vi "102-3102-report5-gaydos.vi"() -> ()   [LabVIEW 2011]
uses:
  <vilib>/imath/engines/lvmath2/RunTimeEngine/ErrorHandling/NIMS_Finalize Error.vi
  <vilib>/imath/engines/lvmath2/RunTimeEngine/Managers/WorkSpace/UID Generator.vi
  <vilib>/imath/engines/lvmath2/RunTimeEngine/Managers/SymbolTable/Clear UID.vi
  <vilib>/imath/engines/lvmath2/RunTimeEngine/NodeEndStatement/NIMS_NodeEndStatement_Output.vi
  <instcachedir>/0/NIMS_NodeEndStatement_Output_53EC0D466D134D7ABD903AC30B43404B.lvgen/NIMS_NodeEndStatement_Output_53EC0D466D134D7ABD903AC30B43404B_005.vi
  <instcachedir>/0/NIMS_NodeEndStatement_Output_53EC0D466D134D7ABD903AC30B43404B.lvgen/NIMS_NodeEndStatement_Output_53EC0D466D134D7ABD903AC30B43404B_000.vi
  <instcachedir>/0/NIMS_NodeEndStatement_Output_53EC0D466D134D7ABD903AC30B43404B.lvgen/NIMS_NodeEndStatement_Output_53EC0D466D134D7ABD903AC30B43404B_001.vi
  <instcachedir>/0/NIMS_NodeEndStatement_Output_53EC0D466D134D7ABD903AC30B43404B.lvgen/NIMS_NodeEndStatement_Output_53EC0D466D134D7ABD903AC30B43404B_004.vi
  <vilib>/imath/engines/lvmath2/RunTimeEngine/RangeToken/NIMS_Range.vi
  <instcachedir>/0/NIMS_Range_0B7635FB69F84E19AA68E7FF959DF37C.lvgen/NIMS_Range_0B7635FB69F84E19AA68E7FF959DF37C_001.vi
  <vilib>/imath/engines/lvmath2/RunTimeEngine/RunTimeType/NIMS_RunTimeType_From StrictType (excl LVString).vi
  <instcachedir>/0/NIMS_RunTimeType_From StrictType (excl LVString)_46AE8B54A11948F0BCCEB8091EE7AA4C.lvgen/NIMS_RunTimeType_From StrictType (excl LVString)_46AE8B54A11948F0BCCEB8091EE7AA4C_000.vi
  <vilib>/imathl/engines/lvmath/Functions/Error Handling/Create Error.vi
  <vilib>/imath/engines/lvmath2/RunTimeEngine/LocalVariableDefStatement/MC_LocalVariableDefStatement_Display.vi
  <vilib>/imath/engines/lvmath2/RunTimeEngine/BuiltInFunctions/zeros/NIMS_V=zeros(I32,I32).vi
  <vilib>/imath/engines/lvmath2/RunTimeEngine/BuiltInFunctions/ones/NIMS_V=ones(I32,I32).vi
  <vilib>/imath/engines/lvmath2/RunTimeEngine/ErrorHandling/NIMS_Create Error From Enums.vi
  <vilib>/imath/engines/lvmath2/RunTimeEngine/BuiltInFunctions/conv/NIMS_conv(V,V).vi
  <instcachedir>/0/NIMS_conv(V,V)_D3E194F2B5174935BB2368CEB7AAC5A9.lvgen/NIMS_conv(V,V)_D3E194F2B5174935BB2368CEB7AAC5A9_000.vi
  <vilib>/imath/engines/lvmath2/RunTimeEngine/ErrorHandling/NIMS_Error From Error Code.vi
  <vilib>/imath/engines/lvmath2/RunTimeEngine/BuiltInFunctions/fft/NIMS_fft(GV).vi
  <instcachedir>/0/NIMS_fft(GV)_4C6467FC22F84E4BA42517A07EF978B0.lvgen/NIMS_fft(GV)_4C6467FC22F84E4BA42517A07EF978B0_000.vi
  <vilib>/imath/engines/lvmath2/RunTimeEngine/BuiltInFunctions/fftshift/NIMS_fftshift(GV).vi
  <instcachedir>/0/NIMS_fftshift(GV)_BD7A7BA9CA6B470B9A9F73A6A3FEEB3E.lvgen/NIMS_fftshift(GV)_BD7A7BA9CA6B470B9A9F73A6A3FEEB3E_000.vi
  <vilib>/imath/engines/lvmath2/RunTimeEngine/ArithmeticOperatorToken/NIMS_ArithmeticOperator_times.vi
  <instcachedir>/0/NIMS_ArithmeticOperator_times_3FA9DDB491BD45F6905798C0465C9825.lvgen/NIMS_ArithmeticOperator_times_3FA9DDB491BD45F6905798C0465C9825_003.vi
  <instcachedir>/0/NIMS_fft(GV)_4C6467FC22F84E4BA42517A07EF978B0.lvgen/NIMS_fft(GV)_4C6467FC22F84E4BA42517A07EF978B0_001.vi
  <vilib>/imath/engines/lvmath2/RunTimeEngine/BuiltInFunctions/ifft_shift/NIMS_ifft_shift(GV).vi
  <instcachedir>/0/NIMS_ifft_shift(GV)_21661D804B78421B969BCA642CA10C0F.lvgen/NIMS_ifft_shift(GV)_21661D804B78421B969BCA642CA10C0F_000.vi
  <vilib>/imath/engines/lvmath2/RunTimeEngine/BuiltInFunctions/ifft/NIMS_ifft(CV).vi
  <vilib>/imath/engines/lvmath2/RunTimeEngine/BuiltInFunctions/length/NIMS_length(GV).vi
  <instcachedir>/0/NIMS_length(GV)_08A3D13377FD4E4B96F5795FBF3698FA.lvgen/NIMS_length(GV)_08A3D13377FD4E4B96F5795FBF3698FA_002.vi
  <vilib>/imath/engines/lvmath2/RunTimeEngine/BuiltInFunctions/abs/NIMS_abs(signed).vi
  <instcachedir>/0/NIMS_abs(signed)_C4FCB8E6058B49B797C7C8D53CA5F6EC.lvgen/NIMS_abs(signed)_C4FCB8E6058B49B797C7C8D53CA5F6EC_006.vi
  <vilib>/imath/engines/lvmath2/RunTimeEngine/BuiltInFunctions/angle/NIMS_angle.vi
  <instcachedir>/0/NIMS_angle_6DDAE2BD99E0421EB990B6436E94D88F.lvgen/NIMS_angle_6DDAE2BD99E0421EB990B6436E94D88F_002.vi
  <vilib>/imath/engines/lvmath2/RunTimeEngine/Managers/SymbolTable/NIMS_WorkSpace.lvlib
panel:
  out "Phase of H(jw)":cluster{"Y":dbl[], "Y":dbl[]}[](graph)
  out "Magnitude of H(jw)":cluster{"Y":dbl[], "Y":dbl[]}[](graph)
  out "Phase of X(jw)":cluster{"Y":dbl[], "Y":dbl[]}[](graph)
  out "Magnitude of X(jw)":cluster{"Y":dbl[], "Y":dbl[]}[](graph)
  out "Phase of Y(jw)":cluster{"Y":dbl[], "Y":dbl[]}[](graph)
  out "Magnitude of Y(jw)":cluster{"Y":dbl[], "Y":dbl[]}[](graph)
  out "y(t) and ift of y(t)":dynamicdata(graph)
  out "h(t)":waveform(dbl)(graph)
  out "x(t)":waveform(i32)(graph)
  in  "D":dbl
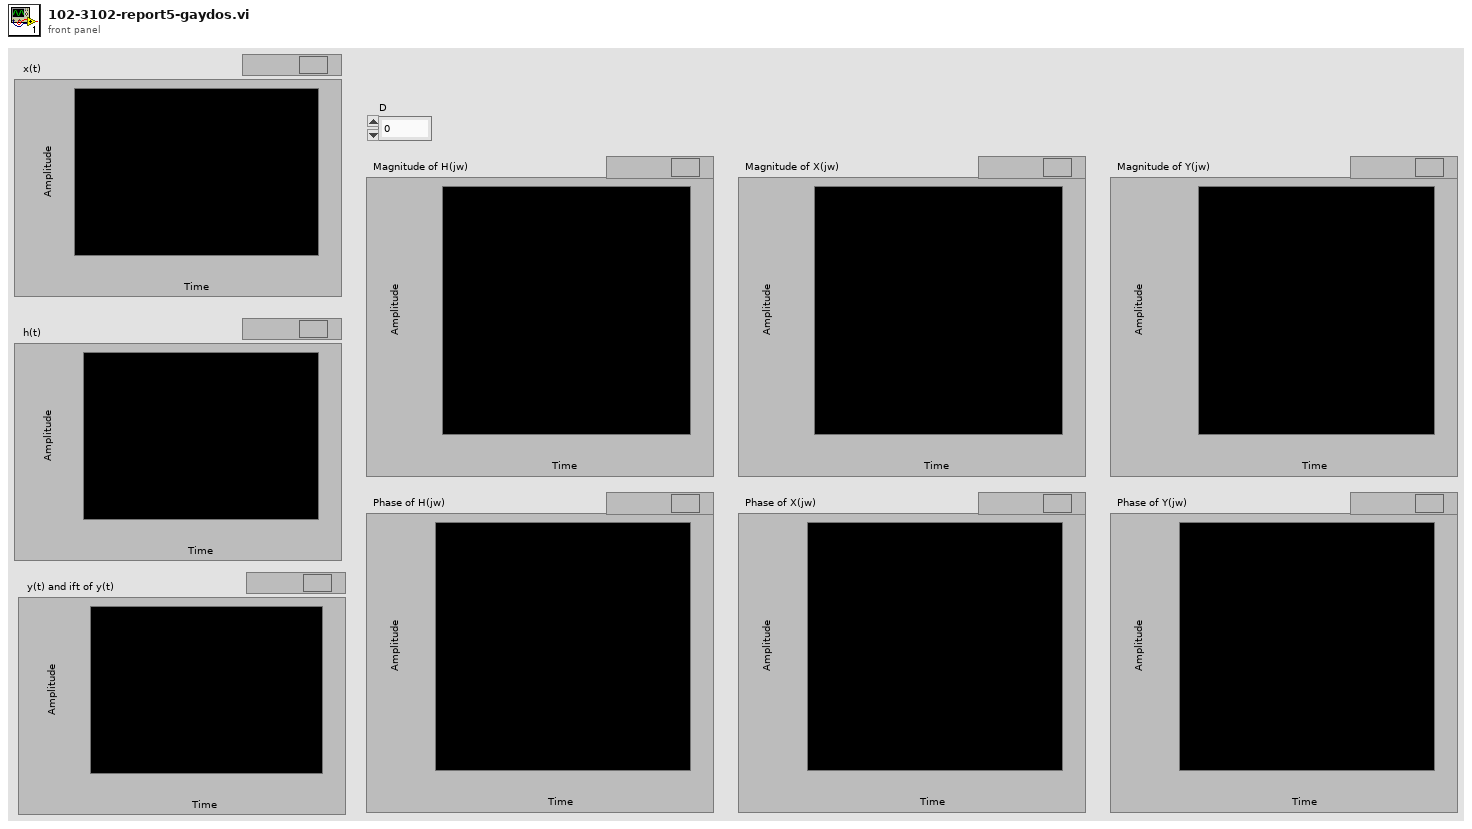
[diagram p1: front panel]
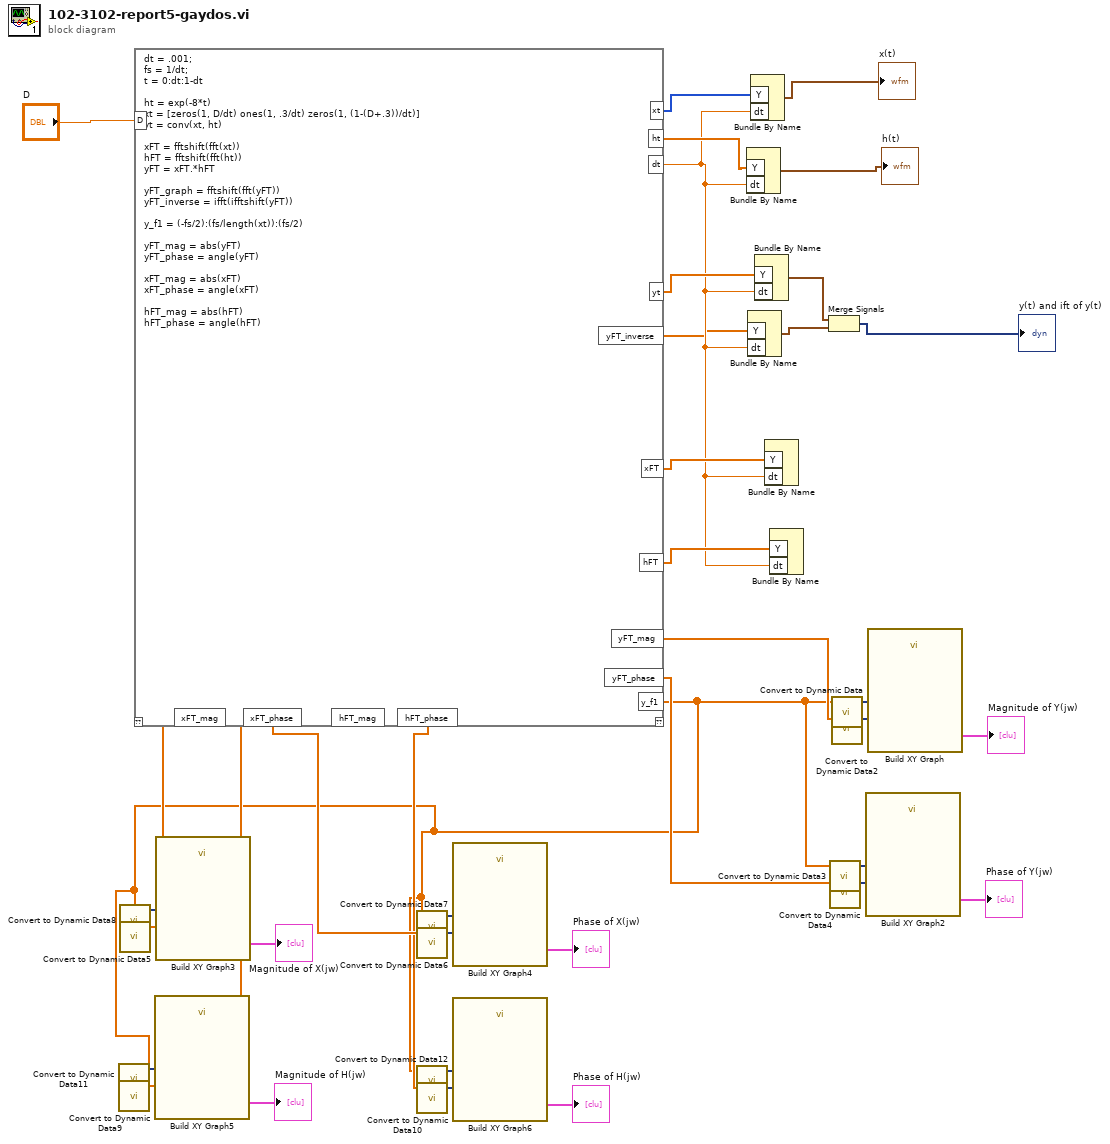
[diagram p0: block diagram]
diagram:
  n1 = mathscript code="dt = .001;\nfs = 1/dt;\nt = 0:dt:1-dt\n\nht = exp(-8*t)\nxt = [zeros(1, D/dt) ones(1, .3/dt) zeros(1, (1-(D+.3))/dt)]\nyt = conv(xt, ht)\n\nxFT = fftshift(fft(xt))\nhFT = fftshift(fft(ht))\nyFT = xFT.*hFT\n\nyFT_graph = fftshift(fft(yFT))\nyFT_inverse = ifft(ifftshift(yFT))\n\ny_f1 = (-fs/2):(fs/length(xt)):(fs/2)\n\nyFT_mag = abs(yFT)\nyFT_phase = angle(yFT)\n\nxFT_mag = abs(xFT)\nxFT_phase = angle(xFT)\n\nhFT_mag = abs(hFT)\nhFT_phase = angle(hFT)"("D"="D") -> ("xt"=w37:i32[], "ht"=w36:dbl[], "dt"=w28:dbl, "yt"=w33:dbl[], "hFT"=w29:cdb[], "xFT"=w30:cdb[], "yFT_mag"=w19:dbl[], "yFT_phase"=w18:dbl[], "yFT_inverse"=w26:dbl[], "y_f1"=w2:dbl[], "xFT_mag"=w15:dbl[], "xFT_phase"=w13:dbl[], "hFT_mag"=w7:dbl[], "hFT_phase"=w5:dbl[])  [unwired: 1 in, 1 out]
  n2 = call "Convert to Dynamic Data11"("Array"=w2) -> ("Dynamic Data Type"=w3:dynamicdata)  [unwired: 3 in]
  n3 = call "Convert to Dynamic Data9"("Array"=w7) -> ("Dynamic Data Type"=w6:dynamicdata)  [unwired: 3 in]
  n4 = call "Convert to Dynamic Data8"("Array"=w2) -> ("Dynamic Data Type"=w10:dynamicdata)  [unwired: 3 in]
  n5 = call "Convert to Dynamic Data5"("Array"=w15) -> ("Dynamic Data Type"=w14:dynamicdata)  [unwired: 3 in]
  n6 = call "Build XY Graph5"("Y Input"=w6, "X Input"=w3) -> ("XY Graph"=→"Magnitude of H(jw)":cluster{"Y":dbl[], "Y":dbl[]}[])  [unwired: 3 in, 6 out]
  n7 = call "Build XY Graph3"("Y Input"=w14, "X Input"=w10) -> ("XY Graph"=→"Magnitude of X(jw)":cluster{"Y":dbl[], "Y":dbl[]}[])  [unwired: 3 in, 6 out]
  n8 = call "Convert to Dynamic Data7"("Array"=w2) -> ("Dynamic Data Type"=w11:dynamicdata)  [unwired: 3 in]
  n9 = call "Convert to Dynamic Data6"("Array"=w13) -> ("Dynamic Data Type"=w12:dynamicdata)  [unwired: 3 in]
  n10 = call "Convert to Dynamic Data12"("Array"=w2) -> ("Dynamic Data Type"=w1:dynamicdata)  [unwired: 3 in]
  n11 = call "Convert to Dynamic Data10"("Array"=w5) -> ("Dynamic Data Type"=w4:dynamicdata)  [unwired: 3 in]
  n12 = call "Build XY Graph4"("Y Input"=w12, "X Input"=w11) -> ("XY Graph"=→"Phase of X(jw)":cluster{"Y":dbl[], "Y":dbl[]}[])  [unwired: 3 in, 6 out]
  n13 = call "Build XY Graph6"("Y Input"=w4, "X Input"=w1) -> ("XY Graph"=→"Phase of H(jw)":cluster{"Y":dbl[], "Y":dbl[]}[])  [unwired: 3 in, 6 out]
  n14 = Bundle By Name("Y"=w36, "dt"=w28) -> (→"h(t)":waveform(dbl))  [unwired: 1 in]
  n15 = Bundle By Name("Y"=w26, "dt"=w28) -> (w25:waveform(dbl))  [unwired: 1 in]
  n16 = Bundle By Name("Y"=w37, "dt"=w28) -> (→"x(t)":waveform(i32))  [unwired: 1 in]
  n17 = Bundle By Name("Y"=w33, "dt"=w28) -> (w32:waveform(dbl))  [unwired: 1 in]
  n18 = Bundle By Name("Y"=w30, "dt"=w28) -> ()  [unwired: 1 in, 1 out]
  n19 = Bundle By Name("Y"=w29, "dt"=w28) -> ()  [unwired: 1 in, 1 out]
  n20 = Merge Signals(w32, w25) -> (→"y(t) and ift of y(t)":dynamicdata)
  n21 = call "Convert to Dynamic Data3"("Array"=w2) -> ("Dynamic Data Type"=w21:dynamicdata)  [unwired: 3 in]
  n22 = call "Convert to Dynamic Data4"("Array"=w18) -> ("Dynamic Data Type"=w20:dynamicdata)  [unwired: 3 in]
  n23 = call "Convert to Dynamic Data"("Array"=w2) -> ("Dynamic Data Type"=w24:dynamicdata)  [unwired: 3 in]
  n24 = call "Convert to Dynamic Data2"("Array"=w19) -> ("Dynamic Data Type"=w23:dynamicdata)  [unwired: 3 in]
  n25 = call "Build XY Graph2"("Y Input"=w20, "X Input"=w21) -> ("XY Graph"=→"Phase of Y(jw)":cluster{"Y":dbl[], "Y":dbl[]}[])  [unwired: 3 in, 6 out]
  n26 = call "Build XY Graph"("Y Input"=w23, "X Input"=w24) -> ("XY Graph"=→"Magnitude of Y(jw)":cluster{"Y":dbl[], "Y":dbl[]}[])  [unwired: 3 in, 6 out]
